vi "Vision Example Robot Main.vi"() -> ()   [LabVIEW 2015]
doc: "This VI implements the framework and scheduler for your robotics program. It should not be necessary to modify the framework. You are expected to add your code to the VIs called from Robot Main - the ones located in the Team Code folder within the project."
uses:
  <vilib>/Rock Robotics/WPI/Camera/WPI_CameraImageSize.ctl
  Robot Global Data.vi
panel:
  in  "Image Size":T1=enum."320x240"
  in  "Enable Vision":bool=TRUE
  in  "Finish":bool
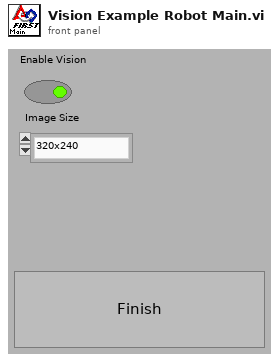
[diagram p1: front panel]
types:
  T1 = typedef "WPI_CameraImageSize.ctl" = enum16{"640x480", "320x240", "160x120", "Custom"}
  T2 = typedef "WPI_DriverStationMatch Info.ctl" = cluster{"Autonomous Elapsed Seconds":dbl, "TeleOp Elapsed Seconds":dbl, "Disabled Elapsed Seconds":dbl, "Visited Autonomous":bool, "Visited TeleOp":bool, "Visited Disabled":bool, "Autonomous Settings":cluster{"Autonomous Style":enum16{"Iterative", "Independent"}, "VI Refnum":refnum<vi>}}
  T3 = typedef "WPI_DriverStationDerivedRobotMode.ctl" = enum16{"Init", "Execute", "Stop"}
  T4 = typedef "WPI_DriverStationRobotMode2.ctl" = enum16{"Autonomous Disabled", "Autonomous Enabled", "Teleop Disabled", "Teleop Enabled", "Disconnected", "Finish", "Test Disabled", "Test Enabled", "Emergency Stopped"}
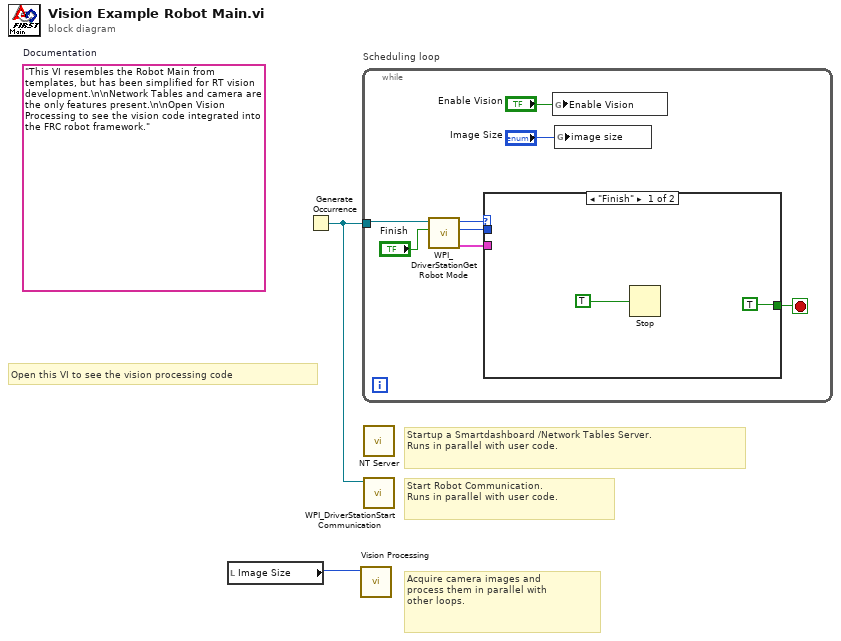
[diagram p0: block diagram]
diagram:
  (unwired) "This VI resembles the Robot Main from templates, but has been simplified for RT vision development.\n\nNetwork Tables and camera are the only features present.\n\nOpen Vision Processing to see the vision code integrated into the FRC robot framework."  # Documentation
  # "Open this VI to see the vision processing code"
  # "Startup a Smartdashboard /Network Tables Server.\nRuns in parallel with user code."
  # "Acquire camera images and\nprocess them in parallel with\nother loops."
  # "Start Robot Communication.\nRuns in parallel with user code."
  n1 = local read "Image Size"() -> (w1:T1)
  n2 = Generate Occurrence() -> (w2:refnum<k4>)
  n3 = call "Vision Processing.vi"("Image Size"=w1) -> ()  [unwired: 1 in, 6 out]
  n4 = while "Scheduling loop" {
    tunnel: w2 -> [w9]
    stop <- w6 stop-if-true
    n5 = call <vilib>:"WPI_DriverStationGet Robot Mode.vi"("Finish"="Finish", "DS Occurrence"=w9) -> ("Match Info out"=w7:T2, "Call Context"=w10:T3, "Robot Mode"=w3:T4)  [unwired: 7 out]
    n6 = case shown="\"Finish\"" w3 {
      tunnel: w10 -> [_ _]
      tunnel: w7 -> [_ _]
      tunnel: [TRUE _] -> w6
      frame "Finish" {
        n7 = Stop(stop? (T)=TRUE ("Quit")) -> ()
      }
      frame Default {
      }
    }
    n8 = global write "Robot Global Data.vi" "Enable Vision"("Enable Vision") -> ()
    n9 = global write "Robot Global Data.vi" "image size"("Image Size") -> ()
  }
  n10 = call <vilib>:"NT Server.vi"() -> ()  [unwired: 12 in]
  n11 = call <vilib>:"WPI_DriverStationStart Communication.vi"("occurrence"=w2) -> ()  [unwired: 1 in, 10 out]
